vi "modbus-to-real.vi"(8 "error in (no error)":errorcluster, 11 "object in":refnum<class "Modbus-Instr.lvclass">) -> (0 "error out":errorcluster, 3 "object out":refnum<class "Modbus-Instr.lvclass">)   [LabVIEW 2021, in "Modbus-Instr.lvclass"]
doc: "Uses adam formula to convert sensors to real No"
uses:
  Modbus-Instr.lvclass
  Modbus-Instr.lvclass/Modbus-Instr.ctl
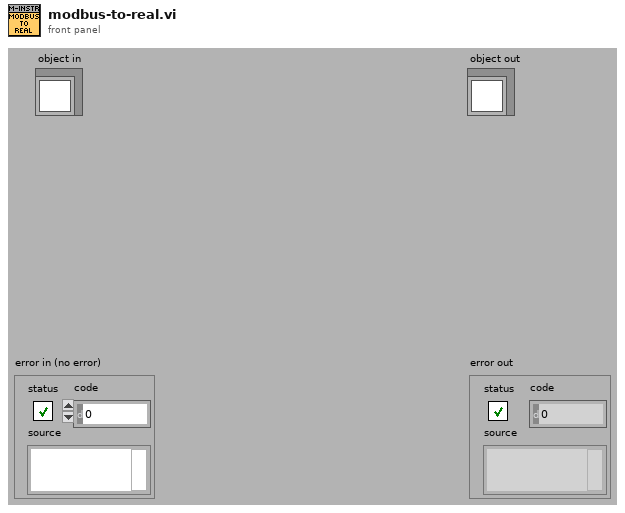
[diagram p1: front panel]
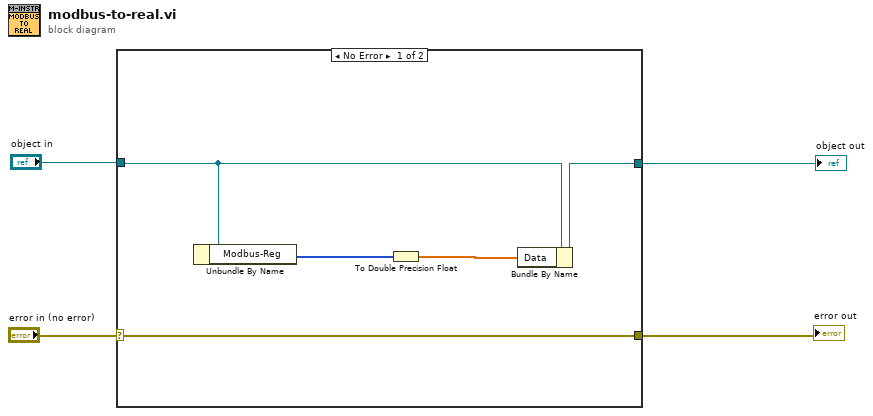
[diagram p0: block diagram]
diagram:
  n1 = case shown="No Error" "error in (no error)" {
    selector: "error in (no error)" -> [w8 w11]
    tunnel: [w8 w11] -> w3
    tunnel: [w6 w10] -> w1
    tunnel: "object in" -> [w7 w10]
    frame No Error {
      n2 = Unbundle By Name(w7) -> ("Modbus-Reg"=w9:u16[])
      n3 = To Double Precision Float(number=w9) -> (double precision float=w5:dbl[])
      n4 = Bundle By Name(cluster=w7, "Data"=w5) -> (w6:refnum<class "Modbus-Instr.lvclass">)
    }
    frame Error {
    }
  }
  "error out" <- w3
  "object out" <- w1
